vi "RELEASE - 2.0 - Motor Control - David G.vi"(3 "Name":string="My Solenoid RefNum", 5 "btnBackward":bool, 7 "btnForward":bool, 8 "FF":dbl=1.0 min=-1.0 max=1.0, 9 "FT":dbl=1.0 min=-1.0 max=1.0, 10 "TF":dbl=1.0 min=-1.0 max=1.0, 11 "TT":dbl=1.0 min=-1.0 max=1.0) -> ()   [LabVIEW 2019]
panel:
  # "TT: Tension au brake\nTF: Vitesse Avant\nFT: Vitesse à reculons\nFF: Tension à l'arrêt"
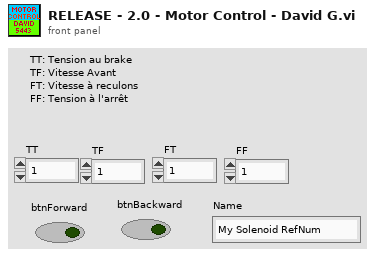
[diagram p1: front panel]
types:
  T1 = typedef "WPI_MotorControlDeviceRef.ctl" = cluster{"DeviceStatus":errorcluster, "Type":T2, "PWM":cluster{"PWM Channel":T3, "DeadBand":T4}, "CAN":cluster{"Device Number":u8, "SetOutput VI Ref":variant, "GetOutput VI Ref":variant, "Enable VI Ref":variant, "Disable VI Ref":variant, "Data":variant}, "Invert":bool, "DIO PWM":cluster{"PWM \"Enable\" Channel":T3, "DIOChannel":T5, "PWM Rate":dbl}}
  T2 = typedef "WPI_MotorControlType.ctl" = enum16{"PWM", "CAN", "DIO PWM"}
  T3 = typedef "FPGA_DIOPWMChannel.ctl" = enum8{"PWM 0", "PWM 1", "PWM 2", "PWM 3", "PWM 4", "PWM 5", "PWM 6", "PWM 7", "PWM 8", "PWM 9", "PWM MXP 0", "PWM MXP 1", "PWM MXP 2", "PWM MXP 3", "PWM MXP 4", "PWM MXP 5", "PWM MXP 6", "PWM MXP 7", "PWM MXP 8", "PWM MXP 9", "Invalid"}
  T4 = typedef "WPI_PWMDeadband.ctl" = cluster{"Name":string, "maxPositivePwm":i32, "minPositivePwm":i32, "centerPwm":i32, "maxNegativePwm":i32, "minNegativePwm":i32, "angularRange":u16}
  T5 = typedef "FPGA_DIOChannel.ctl" = enum8{"DIO 0", "DIO 1", "DIO 2", "DIO 3", "DIO 4", "DIO 5", "DIO 6", "DIO 7", "DIO 8", "DIO 9", "DIO MXP 0", "DIO MXP 1", "DIO MXP 2", "DIO MXP 3", "DIO MXP 4", "DIO MXP 5", "DIO MXP 6", "DIO MXP 7", "DIO MXP 8", "DIO MXP 9", "DIO MXP 10", "DIO MXP 11", "DIO MXP 12", "DIO MXP 13", "DIO MXP 14", "DIO MXP 15", "SPI Port CS1", "SPI Port CS2", "SPI Port CS3", "SPI Port MISO", "SPI Port MOSI", "Invalid"}
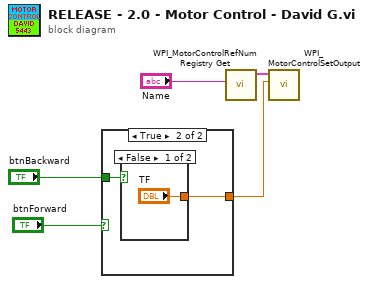
[diagram p0: block diagram]
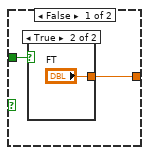
[diagram p2: hidden frame]
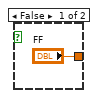
[diagram p3: hidden frame]
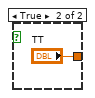
[diagram p4: hidden frame]
diagram:
  n1 = case shown="True" "btnForward" {
    tunnel: "btnBackward" -> [w7 w11]
    tunnel: [w6 w10] -> w1
    frame False {
      n2 = case shown="True" w7 {
        tunnel: ["FF" "FT"] -> w6
        frame False {
        }
        frame True {
        }
      }
    }
    frame True {
      n3 = case shown="False" w11 {
        tunnel: ["TF" "TT"] -> w10
        frame False {
        }
        frame True {
        }
      }
    }
  }
  n4 = call <vilib>:"WPI_MotorControlRefNum Registry Get.vi"("refnum name"="Name") -> ("MotorControlDevRef"=w5:T1)  [unwired: 9 in, 1 out]
  n5 = call <vilib>:"WPI_MotorControlSetOutput.vi"("Output"=w1, "MotorControlDevRef"=w5) -> ()  [unwired: 7 in, 3 out]
